vi "TextLog-Make Entry.vi"(7 "Message":string, 9 "Data":dbl, 11 "error in":errorcluster) -> (15 "error out":errorcluster)   [LabVIEW 2020]
uses:
  TextLog-Queue Data.ctl
  TextLog-Command.ctl
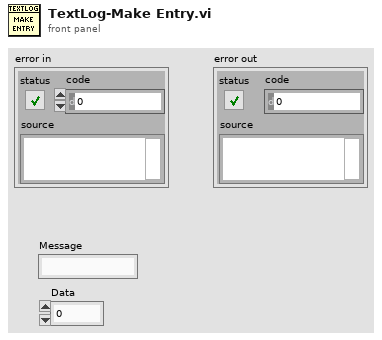
[diagram p1: front panel]
types:
  T1 = typedef "TextLog-Command.ctl" = enum16{"Unspecified", "Start", "Stop", "Quit", "Rename", "Make entry"}
  T2 = typedef "TextLog-Queue Data.ctl" = cluster{"Time":string, "Command":T1, "Message":string, "Data":string}
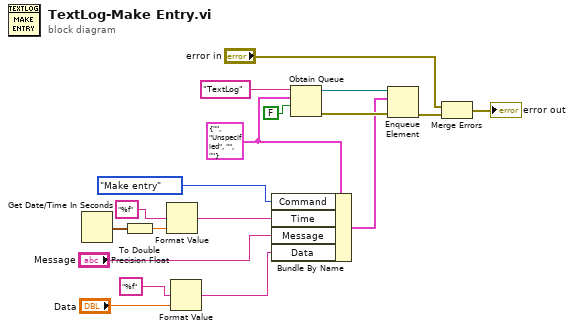
[diagram p0: block diagram]
diagram:
  w16 = T2 {"Time"="", "Command"=enum."Unspecified", "Message"="", "Data"=""} ("Trace Data")
  n1 = Get Date/Time In Seconds() -> (seconds since 1Jan1904=w8:timestamp)
  n2 = To Double Precision Float(number=w8) -> (double precision float=w7:dbl)
  n3 = Format Value(format string="%f", value (0)=w7) -> (output string=w6:string)  [unwired: 1 in]
  n4 = Format Value(format string="%f", value (0)="Data") -> (output string=w2:string)  [unwired: 1 in]
  n5 = Bundle By Name(cluster=w16, "Command"=TextLog-Command."Make entry", "Time"=w6, "Message"="Message", "Data"=w2) -> (w12:T2)
  n6 = Obtain Queue(name (unnamed)="TextLog", element data type=w16, create if not found? (T)=FALSE) -> (queue out=w14:refnum<queue>, error out=w13:errorcluster)  [unwired: 2 in, 1 out]
  n7 = Enqueue Element(queue=w14, element=w12, error in (no error)=w13) -> (error out=w11:errorcluster)  [unwired: 1 in, 2 out]
  n8 = Merge Errors("error in", w11) -> (→"error out":errorcluster)
